vi "Show Hide (Label).vi"(5 "Invert? [F]":bool, 7 "Regex? [F]":bool, 8 "error in (no error)":errorcluster, 9 "Show? [T]":bool=TRUE, 10 "Label":string, 11 "MMI Scaling in":refnum<class "IContainer.lvclass">) -> (0 "error out":errorcluster, 2 "Match?":bool, 3 "MMI Scaling out":refnum<class "IContainer.lvclass">)   [LabVIEW 2013, in "IContainer.lvclass"]
doc: "Copyright 2018, Wiebe Walstra, wiebe@carya.nl."
uses:
  IContainer.lvclass
  IObject.lvclass
  IContainer.lvclass/IContainer.ctl
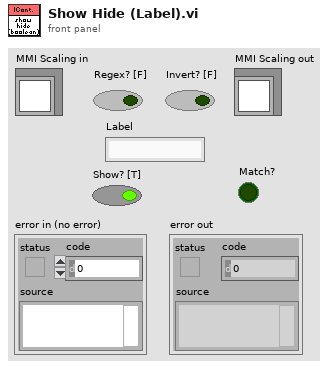
[diagram p1: front panel]
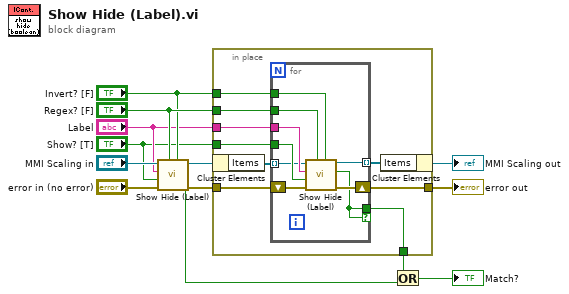
[diagram p0: block diagram]
diagram:
  n1 = call-parent "Show Hide (Label).vi"("Invert? [F]"="Invert? [F]", "Regex? [F]"="Regex? [F]", "error in (no error)"="error in (no error)", "Show? [T]"="Show? [T]", "Label"="Label", "MMI Scaling in"="MMI Scaling in") -> ("error out"=w10:errorcluster, "Match?"=w3:bool, "MMI Scaling out"=w11:refnum<class "IContainer.lvclass">)  [unwired: 3 in]
  n2 = in-place {
    in-place-border: [w22] -> w5
    in-place-border: w10 -> [w21]
    in-place-border: "Show? [T]" -> [w20]
    in-place-border: "Label" -> [w19]
    in-place-border: "Regex? [F]" -> [w16]
    in-place-border: "Invert? [F]" -> [w15]
    in-place-border: [w14] -> w1
    n3 = in-place-cluster #1(w11) -> ("Items"=w18:refnum<class "IObject.lvclass">[])
    n4 = for {
      tunnel: [w30] -> w17 mode=indexing
      tunnel: w18 -> [w24] mode=indexing
      shift-right: [w31] -> w22
      shift-left: w21 -> [w25]
      tunnel: w20 -> [w29]
      tunnel: w19 -> [w28]
      tunnel: w16 -> [w27]
      tunnel: w15 -> [w26]
      tunnel: [w23] -> w14 if=w23
      n5 = call-dynamic "Show Hide (Label).vi"("Invert? [F]"=w26, "Regex? [F]"=w27, "error in (no error)"=w25, "Show? [T]"=w29, "Label"=w28, "MMI Scaling in"=w24) -> ("error out"=w31:errorcluster, "Match?"=w23:bool, "MMI Scaling out"=w30:refnum<class "IObject.lvclass">)  [unwired: 3 in]
    }
    n6 = in-place-cluster #1("Items"=w17) -> (→"MMI Scaling out":refnum<class "IContainer.lvclass">)
  }
  "error out" <- w5
  n7 = Or(x=w1, y=w3) -> (x .or. y?=→"Match?":bool)
